vi "Destroy.vi"(0 "reference in":refnum<class "UI Manager Proxy.lvclass">, 5 "Error In":errorcluster) -> (14 "reference out":refnum<class "UI Manager Proxy.lvclass">, 19 "Error Out":errorcluster)   [LabVIEW 2024, in "UI Manager Proxy.lvclass"]
uses:
  UI Manager Proxy.lvclass
  User Manager_class/User Manager.lvclass
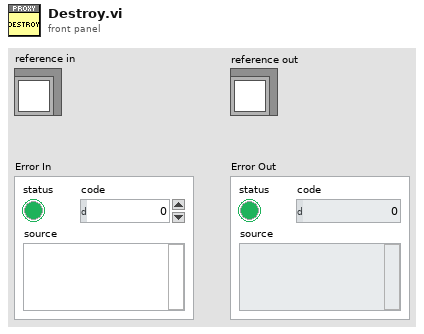
[diagram p1: front panel]
types:
  T1 = typedef "UI Manager Proxy.lvclass/ObjectAttributes.ctl" = cluster{"UI Manager":refnum<class "UI Manager.lvclass">, "UserLevel":T2}
  T2 = typedef "UserLevel.ctl" = enum16{"System Manager", "Admin", "Operator"}
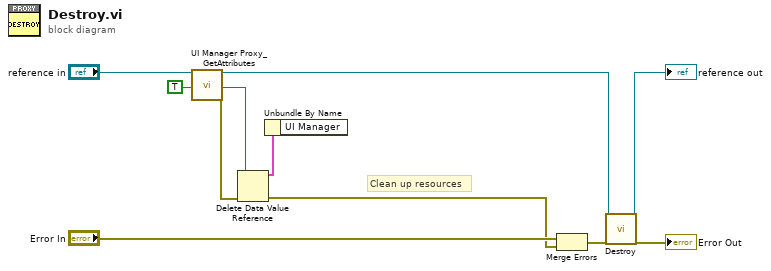
[diagram p0: block diagram]
diagram:
  # "Clean up resources"
  n1 = call "UI Manager Proxy_GetAttributes.vi"("reference in"="reference in", "OnlyGetDvrReference(False)"=TRUE) -> ("reference out"=w6:refnum<class "UI Manager Proxy.lvclass">, "DataRef"=w9:refnum<data-value>, "Error Out"=w10:errorcluster)  [unwired: 14 in, 1 out]
  n2 = Delete Data Value Reference(data value reference=w9, error in=w10) -> (data value=w1:T1, error out=w3:errorcluster)
  n3 = Unbundle By Name(w1) -> ()  [unwired: 1 out]
  n4 = Merge Errors("Error In", w3) -> (w8:errorcluster)
  n5 = call-parent "Destroy.vi"("reference in"=w6, "Error In"=w8) -> ("reference out"=→"reference out":refnum<class "UI Manager Proxy.lvclass">, "Error Out"=→"Error Out":errorcluster)  [unwired: 16 in]
